vi "WLC for dsDNA correction_YCC.vi"() -> ()   [LabVIEW 2014]
uses:
  <vilib>/Utility/file.llb/Read From Spreadsheet File (DBL).vi
  <vilib>/gmath/NumericalOptimization/Nonlinear Curve Fit LM formula string.vi
  <vilib>/Utility/file.llb/Write To Spreadsheet File (DBL).vi
  <vilib>/gmath/NI_Gmath.lvlib
panel:
  out "Force Array  for activated best fit (pN)":dbl[](array[numeric])
  out "Extension array for activated best fit (nm)":dbl[](array[numeric])
  out "Force Array  for unactivated best fit (pN)":dbl[](array[numeric])
  out "Extension array for unactivated best fit (nm)":dbl[](array[numeric])
  in  "Save?":bool
  in  "stop":bool
  in  "file path for unactivated  (dialog if empty)":path=path "D:/YCC/20181219/Success2/195256-F+U--6000.00-5.00-FAh300-raw-U-ForecExtension Only.txt"
  out "Cut-Force for unactivated":dbl[](array[numeric])
  out "Cut-Ex for unactivated":dbl[](array[numeric])
  in  "Tab Control":T1(tab)
  out "F-E curve":cluster{dbl[], dbl[]}(graph)
  out "XY Graph 6":cluster{"best nonlinear fit":dbl[], dbl[]}[](graph)
  out "best fit parameters":dbl[](array[numeric])
  in  "upper bound force (pN)":dbl=30.0
  in  "upper bound extension (nm)":dbl=2000.0
  in  "lower bound force (pN)":dbl=5.0
  in  "lower bound extension (nm)":dbl=400.0
  out "best fit Ex":dbl[](array[numeric])
  out "# of ssDNA nt for unactivated":dbl
  out "dsDNA bp for unactivated(nm)":dbl
  out "F-E curve 2":T2(graph)
  out "Extension for unactivated":dbl[](array[numeric])
  out "Force for unactivated":dbl[](array[numeric])
  # "5180 bp =\n1679+2411=4188 bp dsDNA=\n1002 ssDNA after activated\n\n0.338 nm/bp\n0.56 nm/nt"
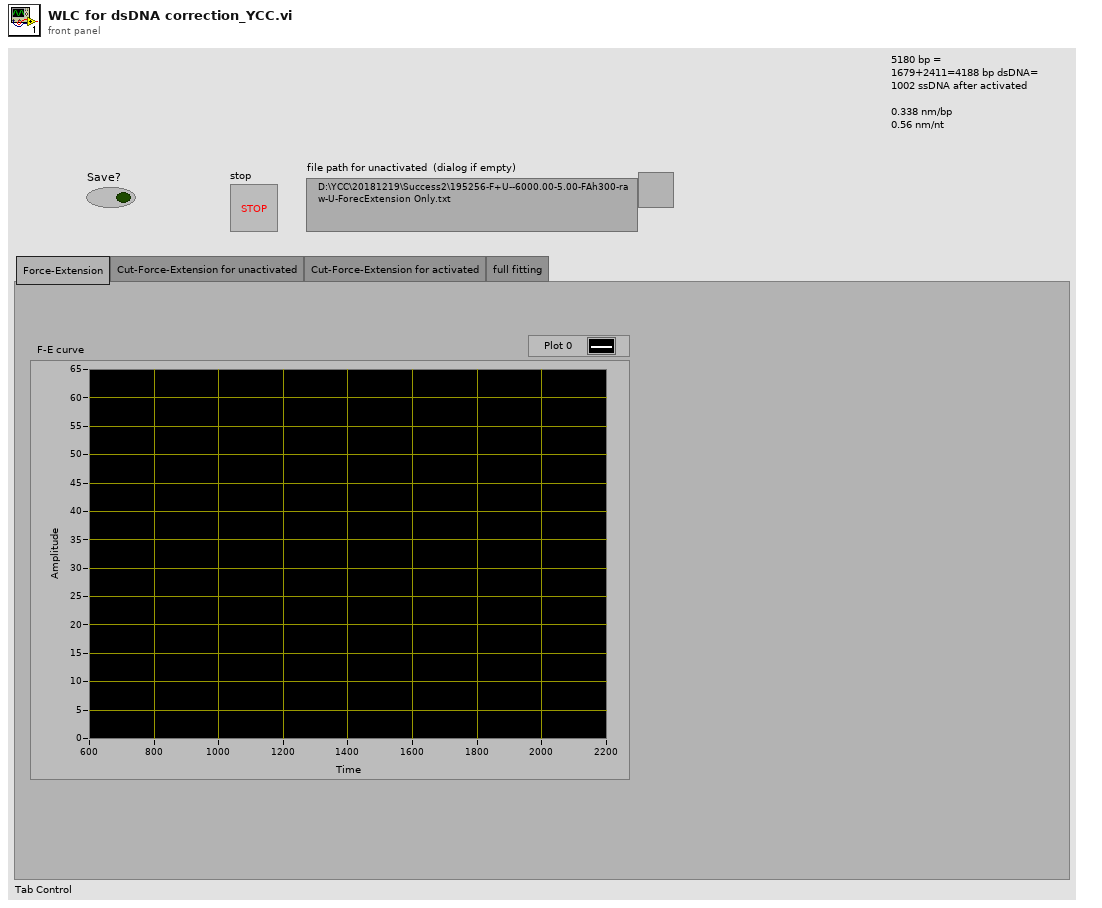
[diagram p1: front panel]
types:
  T1 = enum32{"Force-Extension", "Cut-Force-Extension for unactivated", "Cut-Force-Extension for activated", "full fitting"}
  T2 = cluster{"Extension for unactivated":dbl[], "Force for unactivated":dbl[]}[]
  T3 = cluster{"model":string, "Parameters":string[], "x":string}
  T4 = cluster{"Extension array (nm)":dbl[], "Force Array (pN)":dbl[]}
  T5 = cluster{"Extension for unactivated":dbl[], "Force for unactivated":dbl[]}
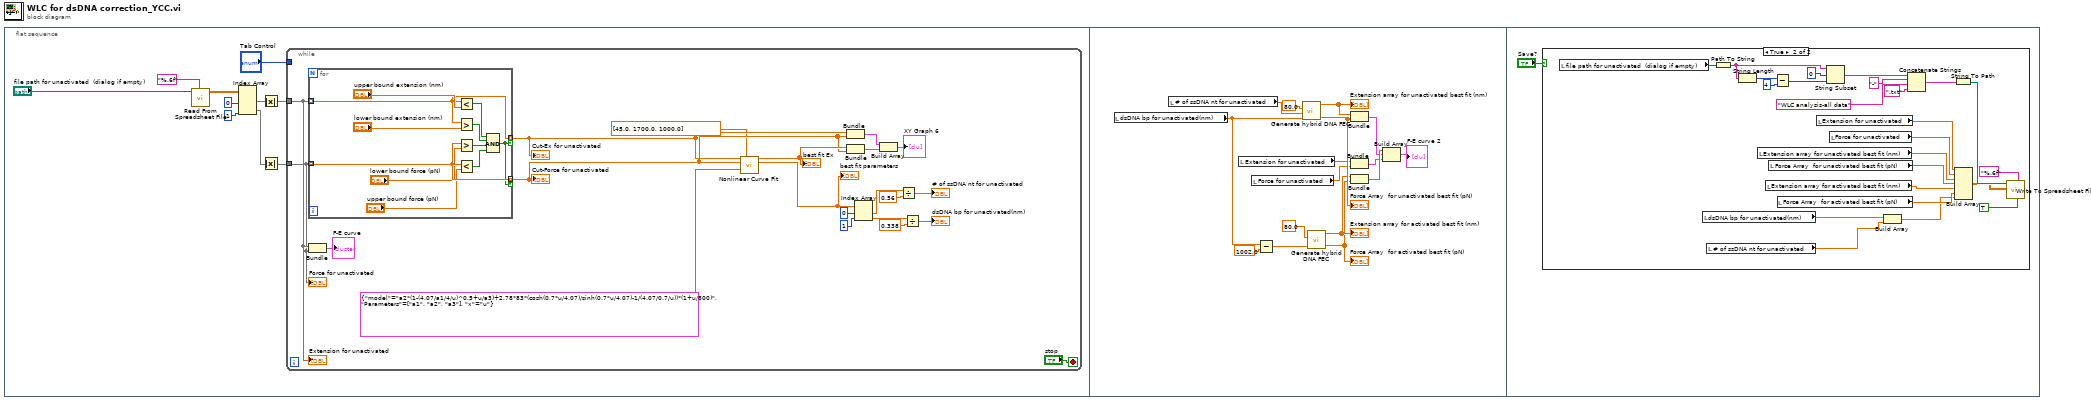
[diagram p0: block diagram]
diagram:
  n1 = flat-sequence {
    frame #0 {
      n2 = call-poly <vilib>:"Read From Spreadsheet File.vi"("format (%.3f)"="%.6f", "file path (dialog if empty)"="file path for unactivated  (dialog if empty)") -> ("all rows"=w1:dbl[][])  [unwired: 5 in, 4 out]
      n3 = Index Array(array=w1, index (col) #1=0 ("disabled index (col)"), index (col) #2=1 ("index (col)")) -> (element #1=w7:dbl[], element #2=w8:dbl[])  [unwired: 2 in]
      n4 = Absolute Value(x=w7) -> (abs(x)=w10:dbl[])
      n5 = Absolute Value(x=w8) -> (abs(x)=w9:dbl[])
      n6 = while {
        tunnel: w10 -> [w23]
        tunnel: w9 -> [w22]
        tunnel: "Tab Control" -> [_]
        stop <- "stop" stop-if-true
        n7 = for {
          tunnel: w22 -> [w42] mode=indexing
          tunnel: [w42] -> w28 mode=indexing if=w40
          tunnel: w23 -> [w35] mode=indexing
          tunnel: [w35] -> w31 mode=indexing if=w40
          n8 = Less?(x=w35, y="upper bound extension (nm)") -> (x < y?=w41:bool)
          n9 = Greater?(x=w35, y="lower bound extension (nm)") -> (0:w34:bool)
          n10 = Greater?(x=w42, y="lower bound force (pN)") -> (0:w33:bool)
          n11 = Less?(x=w42, y="upper bound force (pN)") -> (x < y?=w32:bool)
          n12 = Compound Arithmetic op=AND(w41, w34, w33, w32) -> (w40:bool)
        }
        "Cut-Ex for unactivated" <- w31
        "Cut-Force for unactivated" <- w28
        n13 = Bundle(w23, w22) -> (→"F-E curve":cluster{dbl[], dbl[]})  [unwired: 1 in]
        n14 = call-poly <vilib>:"Nonlinear Curve Fit.vi"("Y"=w31, "initial parameters"=dbl[] [45.0, 1700.0, 1000.0], "X"=w28, "model description"=T3 {"model"="a2*(1-(4.07/a1/4/u)^0.5+u/a3)+2.78*83*(cosh(0.7*u/4.07)/sinh(0.7*u/4.07)-1/(4.07/0.7/u))*(1+u/800)", "Parameters"=["a1", "a2", "a3"], "x"="u"}) -> ("best nonlinear fit"=w29:dbl[], "best fit parameters"=w20:dbl[])  [unwired: 3 in, 7 out]
        "best fit parameters" <- w20
        "best fit Ex" <- w29
        n15 = Bundle(w31, w28) -> (w26:cluster{dbl[], dbl[]})  [unwired: 1 in]
        n16 = Bundle("best nonlinear fit"=w29, w28) -> (w25:cluster{"best nonlinear fit":dbl[], dbl[]})  [unwired: 1 in]
        n17 = Index Array(array=w20, index #1=0 ("index"), index #2=1 ("index")) -> (element #1=w18:dbl, element #2=w12:dbl)
        n18 = Build Array(w26, w25) -> (→"XY Graph 6":cluster{"best nonlinear fit":dbl[], dbl[]}[])
        n19 = Divide(x=w18, y=0.56) -> (x/y=→"# of ssDNA nt for unactivated":dbl)
        n20 = Divide(x=w12, y=0.338) -> (x/y=→"dsDNA bp for unactivated(nm)":dbl)
        "Force for unactivated" <- w22
        "Extension for unactivated" <- w23
      }
    }
    frame #1 {
      n21 = local read "dsDNA bp for unactivated(nm)"() -> (w55:dbl)
      n22 = local read "# of ssDNA nt for unactivated"() -> (w58:dbl)
      n23 = local read "Extension for unactivated"() -> (w50:dbl[])
      n24 = local read "Force for unactivated"() -> (w49:dbl[])
      n25 = Subtract(x=w55, y=1002.0) -> (x-y=w56:dbl)
      n26 = call "Generate hybrid DNA FEC.vi"("End Force (pN)"=80.0, "ssDNA Length (nt)"=w58, "dsDNA Length (bp)"=w55) -> ("Extension array (nm)"=w54:dbl[], "Force Array (pN)"=w53:dbl[])  [unwired: 2 in, 2 out]
      "Extension array for unactivated best fit (nm)" <- w54
      "Force Array  for unactivated best fit (pN)" <- w53
      n27 = call "Generate hybrid DNA FEC.vi"("End Force (pN)"=80.0, "dsDNA Length (bp)"=w56) -> ("Extension array (nm)"=w52:dbl[], "Force Array (pN)"=w51:dbl[])  [unwired: 3 in, 2 out]
      "Extension array for activated best fit (nm)" <- w52
      "Force Array  for activated best fit (pN)" <- w51
      n28 = Bundle("Extension array (nm)"=w54, "Force Array (pN)"=w53) -> (w47:T4)  [unwired: 1 in]
      n29 = Bundle("Extension for unactivated"=w50, "Force for unactivated"=w49) -> (w43:T5)  [unwired: 1 in]
      n30 = Bundle("Extension array (nm)"=w52, "Force Array (pN)"=w51) -> (w48:T4)  [unwired: 1 in]
      n31 = Build Array(w48, w47, w43) -> (→"F-E curve 2":T2)
    }
    frame #2 {
      n32 = case shown="True" "Save?" {
        frame False {
        }
        frame True {
          n33 = local read "file path for unactivated  (dialog if empty)"() -> (w76:path)
          n34 = local read "dsDNA bp for unactivated(nm)"() -> (w64:dbl)
          n35 = local read "# of ssDNA nt for unactivated"() -> (w63:dbl)
          n36 = Path To String(path=w76) -> (string=w71:string)
          n37 = String Length(string=w71) -> (length=w72:i32)
          n38 = local read "Extension array for unactivated best fit (nm)"() -> (w67:dbl[])
          n39 = local read "Extension array for activated best fit (nm)"() -> (w62:dbl[])
          n40 = local read "Force Array  for unactivated best fit (pN)"() -> (w66:dbl[])
          n41 = Subtract(x=w72, y=4) -> (x-y=w75:i32)
          n42 = local read "Force Array  for activated best fit (pN)"() -> (w61:dbl[])
          n43 = local read "Extension for unactivated"() -> (w69:dbl[])
          n44 = String Subset(string=w71, offset (0)=0, length (rest)=w75) -> (substring=w80:string)
          n45 = local read "Force for unactivated"() -> (w68:dbl[])
          n46 = Build Array(w64, w63) -> (w60:dbl[])
          n47 = Concatenate Strings(w80, "-" ("string"), "WLC analysis-all data" ("string"), ".txt" ("string")) -> (w77:string)
          n48 = String To Path(string=w77) -> (path=w70:path)
          n49 = Build Array(w69, w68, w67, w66, w62, w61, w60) -> (w65:dbl[][])
          n50 = call-poly <vilib>:"Write To Spreadsheet File.vi"("transpose? (no:F)"=TRUE, "format (%.3f)"="%.6f", "2D data"=w65, "file path (dialog if empty)"=w70) -> ()  [unwired: 4 in, 1 out]
        }
      }
    }
  }
